vi "Close fd.vi"(8 "error in (no error)":errorcluster, 10 "name of fd":string, 11 "fd":u64) -> (0 "error out":errorcluster)   [LabVIEW 2020, in "NI_Subprocess.lvlib" / "Subprocess.lvclass"]
uses:
  <vilib>/Subprocess/Subprocess/Subprocess.lvclass
  lviosrg.dll
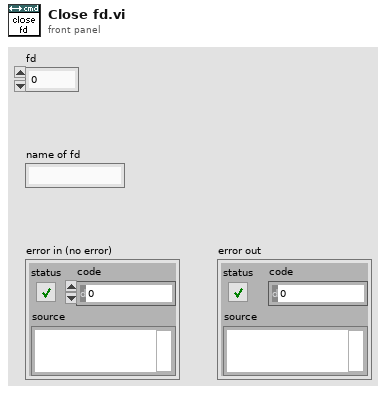
[diagram p1: front panel]
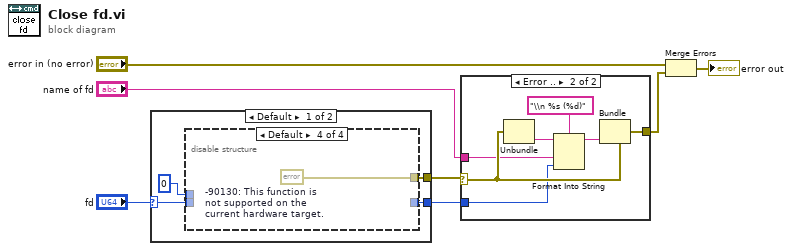
[diagram p0: block diagram]
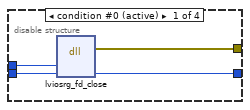
[diagram p3: hidden frame]
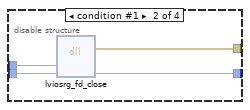
[diagram p4: hidden frame]
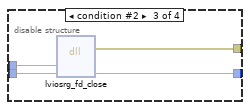
[diagram p5: hidden frame]
diagram:
  n1 = case shown="Default" "fd" {
    selector: "fd" -> [w11 _]
    tunnel: [w9 _] -> w7
    tunnel: [w10 _] -> w6
    frame Default {
      n2 = disable-structure "Conditional Disable Structure" shown="Default" {
        disable-tunnel: w11 -> [w15 w19 w23 _]
        disable-tunnel: [w14 w18 w22 _] -> w10
        disable-tunnel: [w13 w17 w21 w24] -> w9
        disable-tunnel: 0 ("errno") -> [w12 w16 w20 _]
        frame condition #0 (active) {
          n3 = dll-call lib="lviosrg.*" fn="lviosrg_fd_close"("errno"=w12, "fd"=w15) -> (error out=w13:errorcluster, "fd"=w14:u64)  [unwired: 5 in, 1 out]
        }
        frame condition #1 {
          n4 = dll-call lib="lviosrg.*" fn="lviosrg_fd_close"("errno"=w16, "fd"=w19) -> (error out=w17:errorcluster, "fd"=w18:u64)  [unwired: 5 in, 1 out]
        }
        frame condition #2 {
          n5 = dll-call lib="lviosrg.*" fn="lviosrg_fd_close"("errno"=w20, "fd"=w23) -> (error out=w21:errorcluster, "fd"=w22:u64)  [unwired: 5 in, 1 out]
        }
        frame condition #3 {
          w24 = errorcluster {"status"=TRUE, "code"=-90130, "source"=""}  # -90130: This function is not supported on the current hardware target.
        }
      }
    }
    frame 0 {
    }
  }
  n6 = case shown="Error .." w7 {
    selector: w7 -> [w25 w32]
    tunnel: [w25 w28] -> w2
    tunnel: "name of fd" -> [_ w27]
    tunnel: w6 -> [_ w26]
    frame No Error {
    }
    frame Error {
      n7 = Unbundle(w32) -> ("source"=w30:string)  [unwired: 2 out]
      n8 = Format Into String(format string="\\n %s (%d)", initial string=w30, w27, w26) -> (resulting string=w29:string)  [unwired: 1 in, 1 out]
      n9 = Bundle(cluster=w32, "source"=w29) -> (w28:errorcluster)  [unwired: 2 in]
    }
  }
  n10 = Merge Errors("error in (no error)", w2) -> (→"error out":errorcluster)
